vi "SetFloatValue.vi"(1 "error in (no error)":errorcluster, 2 "Float Value":dbl, 3 "Feature Name":string, 4 "IGxDevice":refnum<k24>) -> (0 "error out":errorcluster)   [LabVIEW 2013, in "GxLVlib.lvlib"]
uses:
  GxLVlib.lvlib
  F:/GxILibrary/Labview/trunk/private/dev/src/C#/x64/GxLVLib/dll/GxIAPINET.dll
  private/dev/src/C#/x64/GxLVLib/dll/GxIAPINET.dll
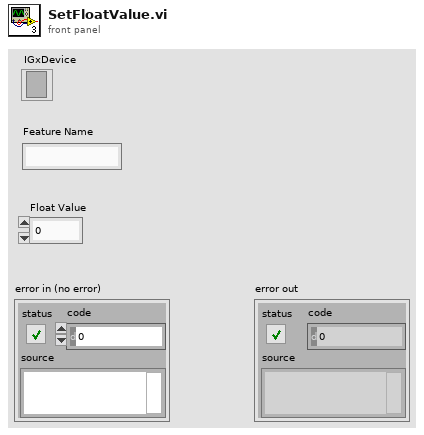
[diagram p1: front panel]
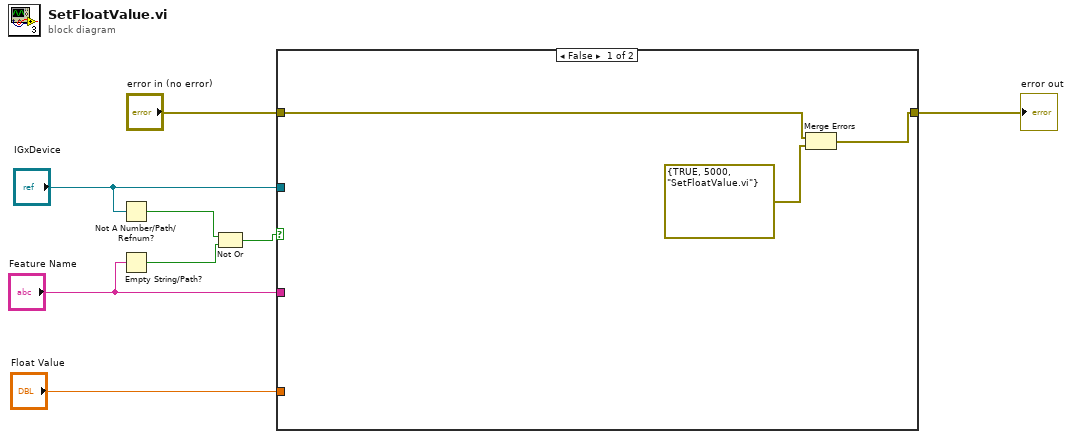
[diagram p0: block diagram]
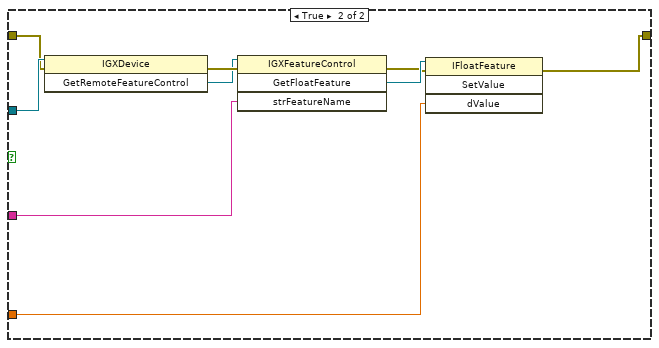
[diagram p2: hidden frame]
diagram:
  n1 = Not A Number/Path/Refnum?(number/path/refnum="IGxDevice") -> (NaN/Path/Refnum?=w8:bool)
  n2 = Empty String/Path?(string/path="Feature Name") -> (empty?=w7:bool)
  n3 = Not Or(1:w7, 2:w8) -> (0:w1:bool)
  n4 = case shown="False" w1 {
    tunnel: "error in (no error)" -> [w10 w19]
    tunnel: [w9 w12] -> w5
    tunnel: "IGxDevice" -> [_ w20]
    tunnel: "Float Value" -> [_ w13]
    tunnel: "Feature Name" -> [_ w16]
    frame False {
      n5 = Merge Errors(w10, errorcluster {TRUE, 5000, "SetFloatValue.vi"}) -> (w9:errorcluster)
    }
    frame True {
      n6 = invoke class="IGXDevice" method="GetRemoteFeatureControl"(reference=w20, error in=w19) -> (error out=w18:errorcluster, "GetRemoteFeatureControl"=w17:refnum<k24>)  [unwired: 1 in, 1 out]
      n7 = invoke class="IGXFeatureControl" method="GetFloatFeature"(reference=w17, error in=w18, "strFeatureName"=w16) -> (error out=w14:errorcluster, "GetFloatFeature"=w15:refnum<k24>)  [unwired: 1 in, 2 out]
      n8 = invoke class="IFloatFeature" method="SetValue"(reference=w15, error in=w14, "dValue"=w13) -> (error out=w12:errorcluster)  [unwired: 1 in, 3 out]
    }
  }
  "error out" <- w5
